vi "Handshake.vi"(8 "error in (no error)":errorcluster, 9 "Timeout (5000ms)":u32=5000, 11 "OpenSSL in":refnum<class "SSL Client Socket.lvclass">) -> (0 "error out":errorcluster, 3 "OpenSSL out":refnum<class "SSL Client Socket.lvclass">)   [LabVIEW 2013, in "OpenSSL Socket.lvlib" / "SSL Client Socket.lvclass"]
uses:
  SSL Client Socket.lvclass
  SSL_Lib/SSL/SSL_Mode.ctl
  Secure Socket/SSL Socket.lvclass/SSL Socket.ctl
  SSL Client Socket.lvclass/SSL Client Socket.ctl
  SSL_Lib/SSL/X509_Host_Verify_Flags.ctl
  Secure Socket/Read BIO.vi
  Read Verify hostname.vi
  Read Server Hostname.vi
  SSL_Lib/BIO/BIO.lvclass
  SSL_Lib/SSL/SSL.lvclass
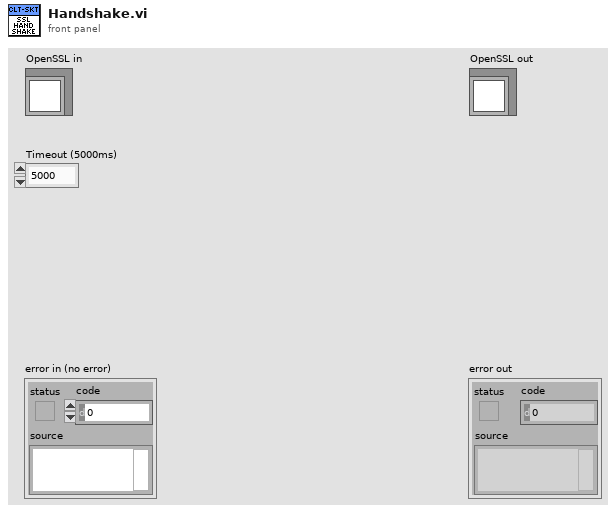
[diagram p1: front panel]
types:
  T1 = typedef "SSL_Lib.lvlib/SSL.lvclass/SSL_Mode.ctl" = i32
  T2 = typedef "SSL_Lib.lvlib/SSL.lvclass/X509_Host_Verify_Flags.ctl" = u32
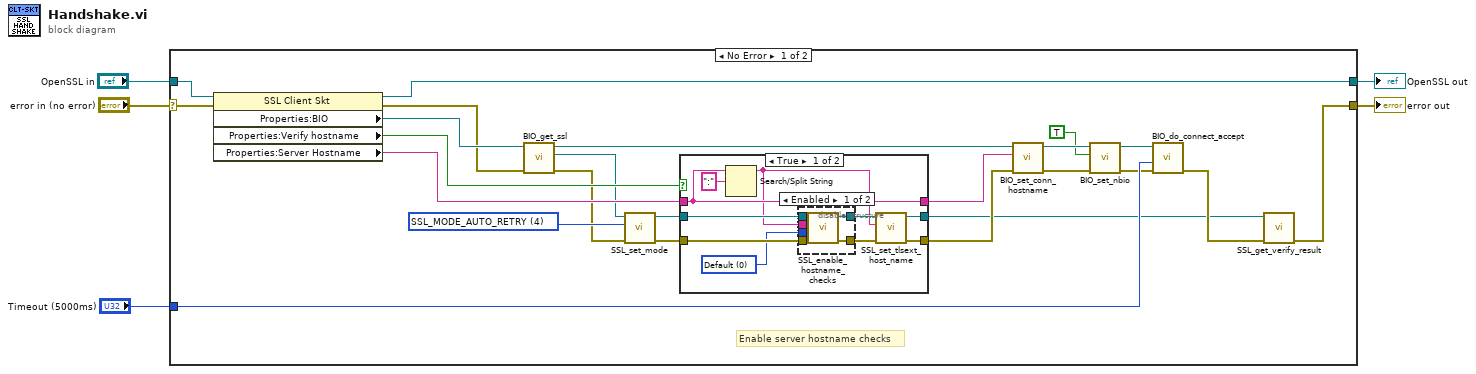
[diagram p0: block diagram]
diagram:
  n1 = case shown="No Error" "error in (no error)" {
    selector: "error in (no error)" -> [w19 w51]
    tunnel: "OpenSSL in" -> [w29 w52]
    tunnel: "Timeout (5000ms)" -> [w25 _]
    tunnel: [w22 w51] -> w3
    tunnel: [w21 w52] -> w2
    frame No Error {
      w10 = T1 4 items=["None"=0, "SSL_MODE_ENABLE_PARTIAL_WRITE"=1, "SSL_MODE_ACCEPT_MOVING_WRITE_BUFFER"=2, "SSL_MODE_AUTO_RETRY"=4, "SSL_MODE_RELEASE_BUFFERS"=16, "SSL_MODE_SEND_FALLBACK_SCSV"=128] ("Mode")
      # "Enable server hostname checks"
      n2 = property class="SSL Client Skt"(reference=w29, error in=w19) -> (reference out=w21:refnum<class "SSL Client Socket.lvclass">, error out=w20:errorcluster, "Properties:BIO"=w23:refnum<class "BIO.lvclass">, "Properties:Verify hostname"=w17:bool, "Properties:Server Hostname"=w16:string)
      n3 = call "BIO_get_ssl.vi"("error in (no error)"=w20, "BIO in"=w23) -> ("error out"=w8:errorcluster, "SSL out"=w9:refnum<class "SSL.lvclass">, "BIO out"=w28:refnum<class "BIO.lvclass">)  [unwired: 7 in]
      n4 = call "SSL_set_mode.vi"("error in (no error)"=w8, "Mode"=w10, "SSL in"=w9) -> ("error out"=w6:errorcluster, "SSL out"=w7:refnum<class "SSL.lvclass">)  [unwired: 7 in]
      n5 = case shown="True" w17 {
        tunnel: w6 -> [w39 w49]
        tunnel: w7 -> [w38 w50]
        tunnel: [w35 w49] -> w27
        tunnel: [w34 w50] -> w24
        tunnel: [w32 w48] -> w18
        tunnel: w16 -> [w32 w48]
        frame True {
          w33 = T2 0 items=["Default"=0, "X509_CHECK_FLAG_ALWAYS_CHECK_SUBJECT"=1, "X509_CHECK_FLAG_NO_WILDCARDS"=2, "X509_CHECK_FLAG_NO_PARTIAL_WILDCARDS"=4, "X509_CHECK_FLAG_MULTI_LABEL_WILDCARDS"=8, "X509_CHECK_FLAG_SINGLE_LABEL_SUBDOMAINS"=16] ("Verification Flags")
          n6 = Search/Split String(string=w32, search string/char (-)=":") -> (substring before match=w30:string)  [unwired: 1 in, 2 out]
          n7 = disable-structure shown="Enabled" {
            disable-tunnel: w39 -> [w45 w46]
            disable-tunnel: w38 -> [w44 w47]
            disable-tunnel: [w43 w47] -> w37
            disable-tunnel: [w42 w46] -> w36
            disable-tunnel: w33 -> [w41 _]
            disable-tunnel: w30 -> [w40 _]
            frame Enabled {
              n8 = call "SSL_enable_hostname_checks.vi"("error in (no error)"=w45, "Verification Flags"=w41, "Hostname"=w40, "SSL in"=w44) -> ("error out"=w42:errorcluster, "SSL out"=w43:refnum<class "SSL.lvclass">)  [unwired: 6 in]
            }
            frame Disabled {
            }
          }
          n9 = call "SSL_set_tlsext_host_name.vi"("error in (no error)"=w36, "Hostname"=w30, "SSL in"=w37) -> ("error out"=w35:errorcluster, "SSL out"=w34:refnum<class "SSL.lvclass">)  [unwired: 7 in]
        }
        frame False {
        }
      }
      n10 = call "BIO_set_conn_hostname.vi"("error in (no error)"=w27, "Hostname"=w18, "BIO in"=w28) -> ("error out"=w14:errorcluster, "BIO out"=w15:refnum<class "BIO.lvclass">)  [unwired: 7 in]
      n11 = call "BIO_set_nbio.vi"("error in (no error)"=w14, "Non-Blocking?"=TRUE, "BIO in"=w15) -> ("error out"=w13:errorcluster, "BIO out"=w12:refnum<class "BIO.lvclass">)  [unwired: 7 in]
      n12 = call "BIO_do_connect_accept.vi"("error in (no error)"=w13, "Timeout (10000ms)"=w25, "BIO in"=w12) -> ("error out"=w26:errorcluster)  [unwired: 7 in, 1 out]
      n13 = call "SSL_get_verify_result.vi"("error in (no error)"=w26, "SSL-Lib in"=w24) -> ("error out"=w22:errorcluster)  [unwired: 7 in, 2 out]
    }
    frame Error {
    }
  }
  "error out" <- w3
  "OpenSSL out" <- w2
